vi "HatchRect.vi"() -> ()   [LabVIEW 2014]
uses:
  TypeDefs/Point2DwSlope.ctl
panel:
  out "Combined":T2
  out "XY Graph":cluster{"X":sgl, "Y":sgl, "Slope":dbl}[](graph)
  in  "Angle":sgl=45.0
  in  "Height":dbl=2.0 format="%#_13g"
  in  "Width":dbl=1.0 format="%#_13g"
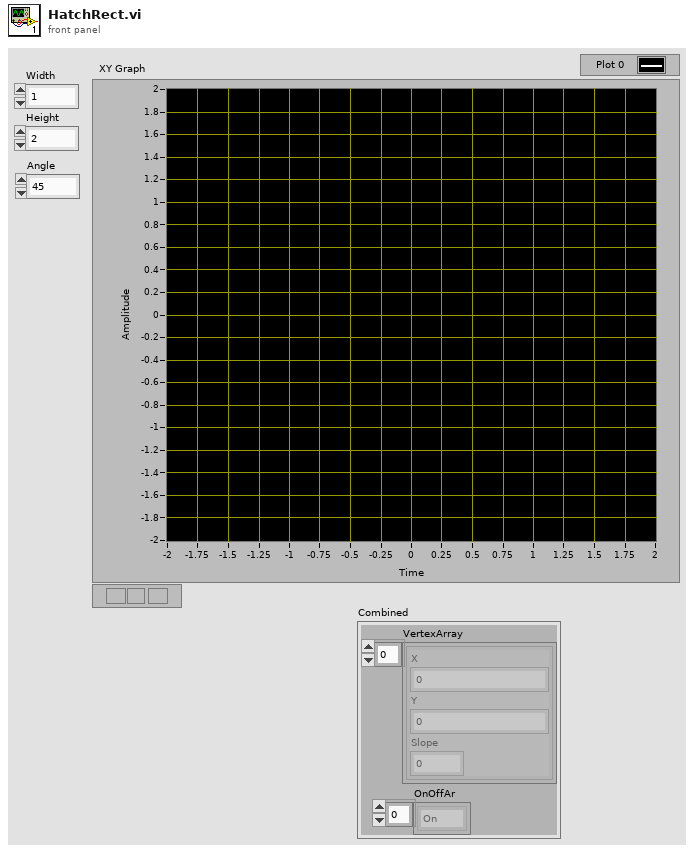
[diagram p1: front panel]
types:
  T1 = typedef "Point2DwSlope.ctl" = cluster{"X":sgl, "Y":sgl, "Slope":dbl}
  T2 = cluster{"VertexArray":T1[], "OnOffAr":enum16{"On", "Off"}[]}
  T3 = cluster{"Xmin":dbl, "Xmax":dbl, "Ymin":dbl, "Ymax":dbl}
  T4 = typedef "Poly2DwSlope.ctl" = cluster{"VertexArray":T1[]}
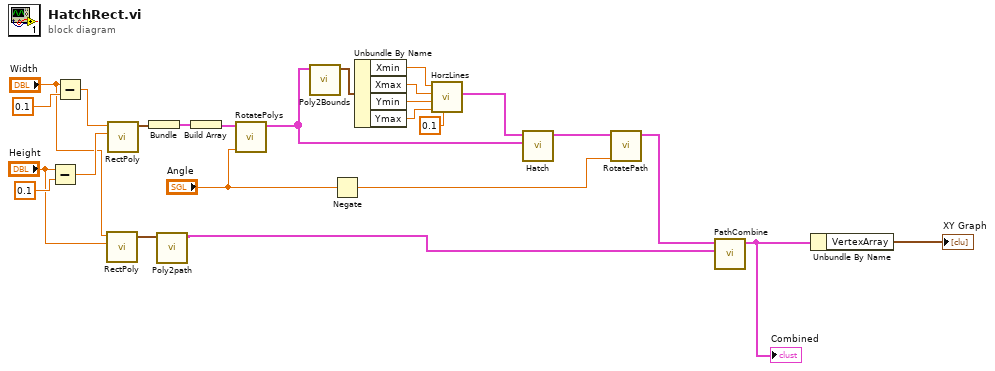
[diagram p0: block diagram]
diagram:
  n1 = Subtract(x="Height", y=0.1) -> (x-y=w7:dbl)
  n2 = Subtract(x="Width", y=0.1) -> (x-y=w8:dbl)
  n3 = call "RectPoly.vi"("Height"="Height", "Width"="Width") -> ("VertexArray"=w5:T1[])  [unwired: 9 in]
  n4 = call "RectPoly.vi"("Height"=w7, "Width"=w8) -> ("VertexArray"=w25:T1[])  [unwired: 9 in]
  n5 = Bundle("VertexArray"=w25) -> (w24:cluster{"VertexArray":T1[]})  [unwired: 1 in]
  n6 = call "Poly2path.vi"("VertexArray"=w5) -> ("Path"=w4:T2)  [unwired: 10 in]
  n7 = Build Array(w24) -> (w16:cluster{"VertexArray":T1[]}[])
  n8 = call "RotatePolys.vi"("Angle"="Angle", "Polys"=w16) -> ("RotatedPolys"=w15:cluster{cluster{sgl, sgl, "Slope":dbl}[]}[])  [unwired: 9 in]
  n9 = call "Poly2Bounds.vi"("Polys"=w15) -> ("Bounds"=w23:T3)  [unwired: 10 in]
  n10 = Negate(x="Angle") -> (-x=w12:sgl)
  n11 = Unbundle By Name(w23) -> ("Xmin"=w22:dbl, "Xmax"=w21:dbl, "Ymin"=w20:dbl, "Ymax"=w19:dbl)
  n12 = call "HorzLines.vi"("Spacing"=0.1, "yMax"=w19, "yMin"=w20, "xMax"=w21, "xMin"=w22) -> ("Poly2D"=w18:T4)  [unwired: 5 in, 1 out]
  n13 = call "Hatch.vi"("Polys"=w15, "Hatch"=w18) -> ("Path"=w14:T2)  [unwired: 9 in]
  n14 = call "RotatePath.vi"("Angle"=w12, "Path"=w14) -> ("RotatedPath"=w6:T2)  [unwired: 9 in]
  n15 = call "PathCombine.vi"("Path2"=w4, "Path1"=w6) -> ("Combined"=w3:T2)  [unwired: 9 in]
  "Combined" <- w3
  n16 = Unbundle By Name(w3) -> ("VertexArray"=→"XY Graph":T1[])
